vi "start_leds.vi"(8 "ERROR IN":errorcluster, 10 "notifier out":refnum<notifier>, 11 "LED THREAD":refnum<queue>) -> (0 "error out":errorcluster, 3 "LED THREAD OUT":refnum<queue>)   [LabVIEW 2013]
uses:
  main_machine/type_defs/led_mm.ctl
  main_machine/type_defs/global_settings.ctl
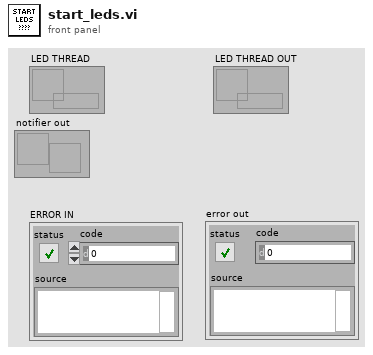
[diagram p1: front panel]
types:
  T1 = typedef "global_settings.ctl" = cluster{"# REACTORS":u32, "17X PORT":i32, "WASTE POSITION ":i32, "SECONDS BETWEEN SAMPLING":dbl, "FACS DIVA DIRECTORY":path, "DATA FILE":path, "REACTORS TO USE":u32[], "PULSE PERIOD":i32, "USE LIGHTS?":bool, "LED FILE":path, "LED CHANNELS":u32[], "PULSE LENGTH":i32, "SUMMARY FILE":path, "OUTGROWTH TIME POINTS":dbl, "SELECTION VALVE PORT":refnum<visa-resource-name>, "HTS PORT":refnum<visa-resource-name>, "DILUTION VOLUME (uL)":i32, "DILUTION FILE":path, "1X PORT":i32}
  T2 = typedef "led_mm.ctl" = enum16{"INITALIZE", "START LEDS", "STROBE", "SHUTDOWN"}
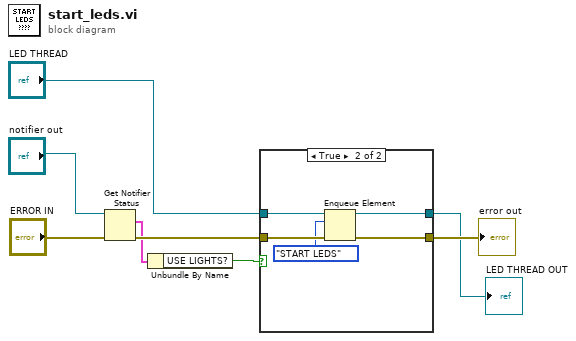
[diagram p0: block diagram]
diagram:
  n1 = Get Notifier Status(notifier="notifier out", error in (no error)="ERROR IN") -> (current notification=w2:T1, error out=w8:errorcluster)  [unwired: 3 out]
  n2 = Unbundle By Name(w2) -> ("USE LIGHTS?"=w1:bool)
  n3 = case shown="True" w1 {
    tunnel: w8 -> [w9 w15]
    tunnel: "LED THREAD" -> [w10 w14]
    tunnel: [w10 w13] -> w4
    tunnel: [w9 w11] -> w5
    frame False {
    }
    frame True {
      n4 = Enqueue Element(queue=w14, element=led_mm."START LEDS", error in (no error)=w15) -> (queue out=w13:refnum<queue>, error out=w11:errorcluster)  [unwired: 1 in, 1 out]
    }
  }
  "LED THREAD OUT" <- w4
  "error out" <- w5
